vi "NI 5772 (AC) Digitizer(FPGA).vi"() -> ()   [LabVIEW 2020]
doc: "Example Description:\nThis example demonstrates how to enable Time Interleaved Sampling with the NI 5772 adapter module to achieve a sampling rate of 1.6GS/s. This example continuously acquires records of analog input data from the NI 5772 adapter module. It allows you to select an AI channel, trigger type, and record size. This VI must be compiled before it is run. \n\nRunning the VI:\nThis VI must be run from the NI 5772 - Getting Started (Host).vi. Refer to the host VI documentation for steps regarding running and configuring the FPGA VI. \n\nExecution Steps:\nRefer to the Block Diagram of this VI for execution comments."
uses:
  Controls/AI Trigger Type.ctl
  Controls/Aquire State.ctl
  <vilib>/Platform/TimedLoop/XDataNode/timing_clust.ctl
  <vilib>/Platform/TimedLoop/XDataNode/nitl_modes.ctl
  <vilib>/Platform/TimedLoop/XDataNode/wakeup.ctl
  Controls/DigitizerState.ctl
  <instrlib>/_niInstr/Data Trigger/v1/Shared/Public/Edge Configuration Bool.ctl
  <instrlib>/_niInstr/Data Trigger/v1/Shared/Public/Edge Configuration Trigger Slope.ctl
  <vilib>/rvi/Emulation/niFpgaGetClockAttributes.vi
  <vilib>/rvi/Emulation/niFpgaSctlEmulationGetInTimedLoop.vi
  <vilib>/rvi/Emulation/niFpgaEmulationReportErrorSimple.vi
  <vilib>/rvi/eio/common/nirviEmuTemplateMethod_errors.vi
  <vilib>/rvi/Emulation/niFpgaCriticalErrorInLSC.vi
  <instrlib>/_niInstr/Data Trigger/v1/FPGA/Private/Trigger/Edge Boolx1spc.vi
  <vilib>/rvi/Emulation/niFpgaEmulationIsFPGAContextNoSignature.vi
  <vilib>/rvi/errors/niFpgaSetErrorForExecOnDevCompSimple.vi
  <vilib>/rvi/eio/common/nirviEmuReportErrorAndStop.vi
  <vilib>/rvi/DataTransferAndStorage/Container/Common/niFpgaContainerGetUniqueNameForEmu.vi
  <vilib>/rvi/FIFO/Fifo_Resource/nirvififoEmulationSetSize.vi
  <vilib>/rvi/FIFO/Fifo_Resource/nirviFifoEmulationQueueMgr.vi
  <instcachedir>/0/nirviFifoEmulationQueueMgr_E5CAEC123FF24DC58D834DCA3CDAA9B5.lvgen/nirviFifoEmulationQueueMgr_E5CAEC123FF24DC58D834DCA3CDAA9B5_000.vi
  <vilib>/rvi/FIFO/Fifo_Resource/nirvififoEmulationDetermineInputValidOut.vi
  <vilib>/rvi/FIFO/Fifo_Resource/nirvififoEmulationCreateLock.vi
  <vilib>/rvi/Emulation/niFpgaProcessEmulError.vi
  <vilib>/rvi/FIFO/Fifo_Resource/nirvififoEmulationObtainLock.vi
  <vilib>/rvi/FIFO/Fifo_Resource/nirvififoEmulationReleaseLock.vi
  <vilib>/rvi/occurrence/nirviWaitOnOccurrenceBase.vi
  <vilib>/rvi/errors/nirviReportUnexpectedCaseInternalError.vi
  <vilib>/rvi/errors/nirviReportUnexpectedCaseInternalError (U32).vi
  <vilib>/Utility/error.llb/Clear Errors.vi
  <instcachedir>/0/nirviFifoEmulationQueueMgr_E5CAEC123FF24DC58D834DCA3CDAA9B5.lvgen/nirviFifoEmulationQueueMgr_E5CAEC123FF24DC58D834DCA3CDAA9B5_003.vi
  <vilib>/rvi/interface/RandomDataEmulation/niFpgaRandomDataHandleErrors.vi
  <vilib>/eio/EIONode/EIONode.xnode
  <vilib>/Platform/TimedLoop/XDataNode/XDataNode.xnode
  <vilib>/rvi/DataTransferAndStorage/Container/XNode/niFpgaContainer.xnode
  <vilib>/rvi/FIFO/Fifo_Resource/nirvififoEmulationWrite.vi
  <vilib>/rvi/FIFO/Fifo_Resource/nirvififoEmulationRead.vi
  <vilib>/rvi/FIFO/Fifo_Resource/nirvififoEmulationGetNumberOfElementsToRead.vi
  <vilib>/Platform/TimedLoop/XDataNode/XDNodeRunTimeDep.lvlib
  <instrlib>/_niInstr/Data Trigger/v1/FPGA/niInstr Data Trigger v1 FPGA.lvlib
  <instrlib>/_niInstr/Data Trigger/v1/Shared/niInstr Data Trigger v1 Shared.lvlib
  <vilib>/rvi/interface/RandomDataEmulation/nirviRandomDataFpgaReadWriteTemplate.vi
panel:
  out "DMA FIFO Overflow?":bool caption="FIFO Overflow?"
  in  "AvgCount":u16=1
  out "Avg FIFO Overflow?":bool caption="FIFO Overflow?"
  in  "vi/nGenTrig":bool
  in  "TrigIn Simulate":bool
  in  "Delay after Trig [cycles]":u16
  out "TS FIFO In Overflow?":bool caption="FIFO Overflow?"
  in  "Quad Samples Per Trigger":u16=512 caption="Samples Per Trigger" min=1 step=1
  in  "Arm Trigger":bool
  in  "User Command Commit":bool
  in  "User Command":u8
  out "User Command Idle":bool
  out "User Command Status":u8
  in  "User Data 0":u16
  in  "User Data 1":u8
  out "PLL Locked":bool
  out "User Error":bool
  out "Configured?":bool
  in  "Trigger Level":i16
  in  "Trigger Type":T1
  # "Resource Configuration"
  # "Analog Input"
  # "Clock Configuration"
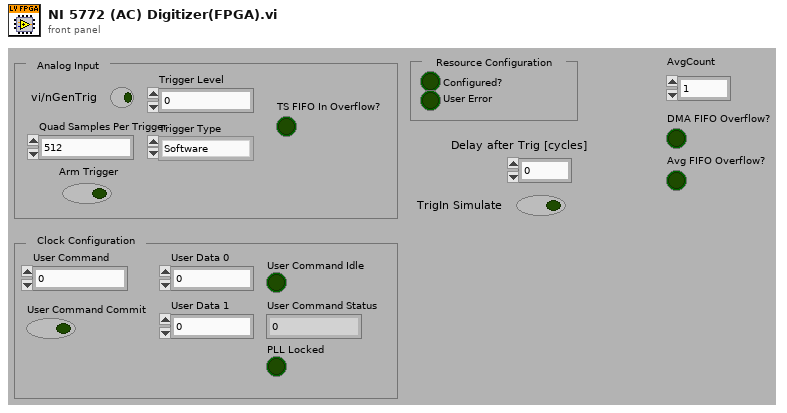
[diagram p1: front panel]
types:
  T1 = typedef "AI Trigger Type.ctl" = enum8{"Software", "Data Edge"}
  T2 = typedef "DigitizerState.ctl" = enum16{"GetData", "Filter", "AverageCountCheck", "SendtoHost", "CompleteScan"}
  T3 = typedef "Aquire State.ctl" = enum8{"Idle", "Wait for Trigger", "Hold Aquire", "Acquire"}
  T4 = typedef "XDNodeRunTimeDep.lvlib/timing_clust.ctl" = cluster{"Expected End [f-1]":u64, "Actual End [f-1]":u64, "Finished Late? [f-1]":bool, "Expected End [i-1]":u64, "Actual End [i-1]":u64, "Finished Late? [i-1]":bool, "Expected Start [i]":u64, "Actual Start [i]":u64, "Expected Start [f]":u64, "Actual Start [f]":u64, "Source Name":string, "Structure Name":string, "Period":i64, "Deadline":i64, "Offset":i64, "Start":i64, "Priority":i32, "Timeout":i32, "Mode":T5, "Wakeup Reason":T6, "Error":errorcluster, "Source Type":string, "Secondary Source Type":string, "Global End Time":u64, "Global Start Time":u64, "Frame Duration":u64, "Iteration Duration":u64, "Assigned CPU":i32, "I/O Scan Engine Mode":u32}
  T5 = typedef "XDNodeRunTimeDep.lvlib/nitl_modes.ctl" = enum32{"No Change", "Process missed periods, maintain original phase", "Discard missed periods, maintain original phase", "Process missed periods, ignore original phase", "Discard missed periods, ignore original phase"}
  T6 = typedef "XDNodeRunTimeDep.lvlib/wakeup.ctl" = enum32{"Normal", "Aborted", "Asynchronous wakeup", "Timing source error", "Timed loop error", "Timeout"}
  T7 = typedef "niInstr Data Trigger v1 Shared.lvlib/Edge Configuration Bool.ctl" = cluster{"trigger slope":T8}
  T8 = typedef "niInstr Data Trigger v1 Shared.lvlib/Edge Configuration Trigger Slope.ctl" = enum8{"Positive", "Negative"}
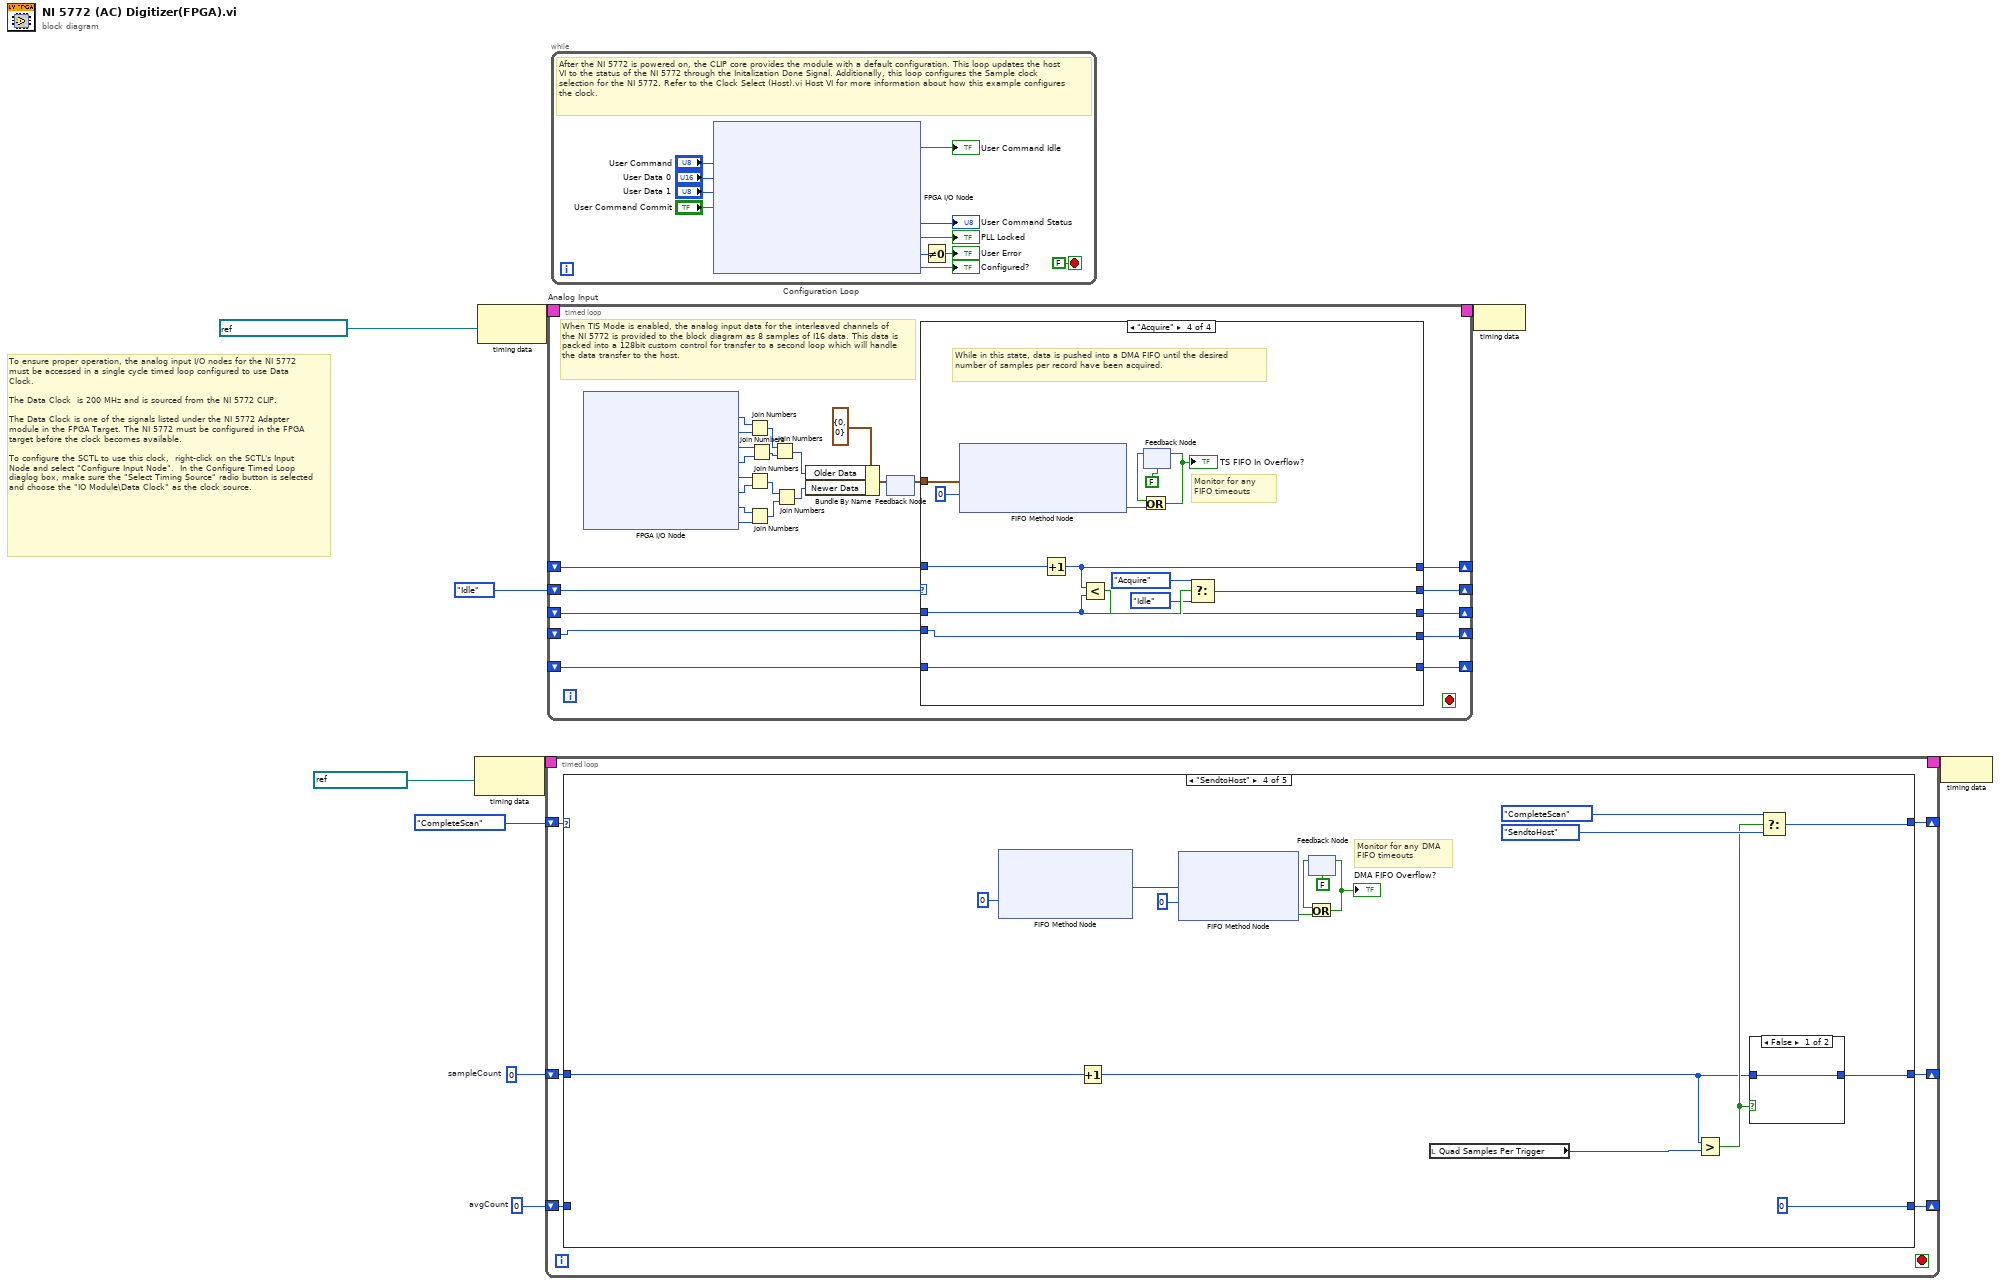
[diagram p0: block diagram]
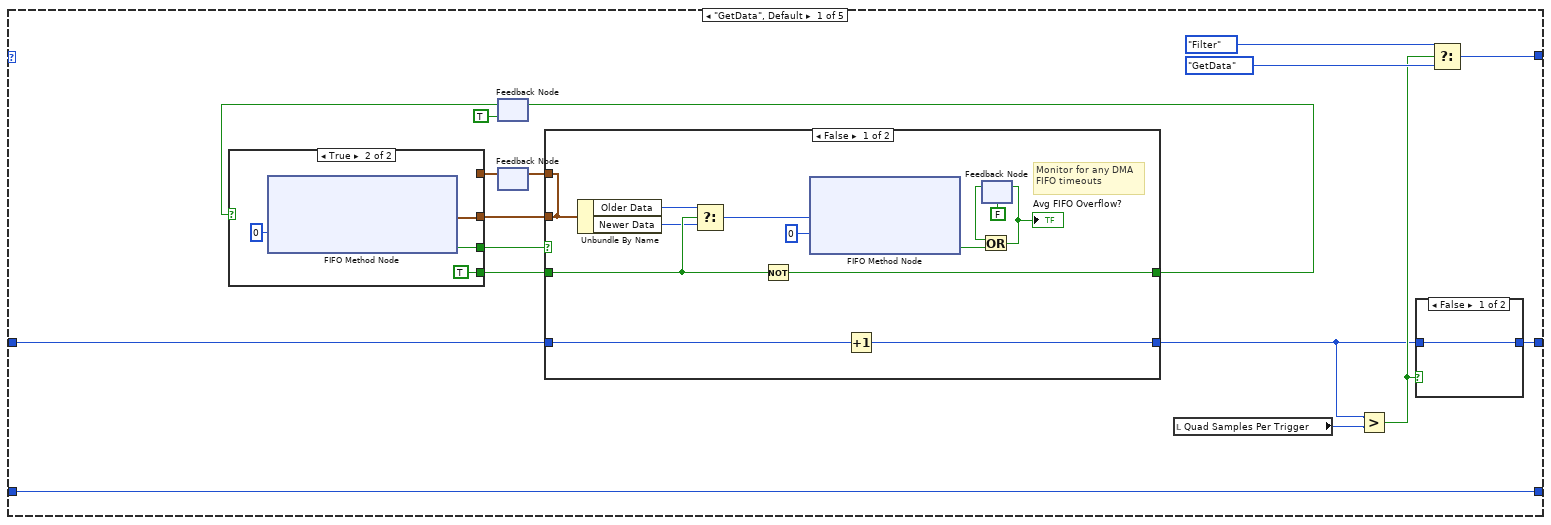
[diagram p2: hidden frame]
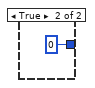
[diagram p3: hidden frame]
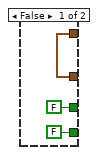
[diagram p4: hidden frame]
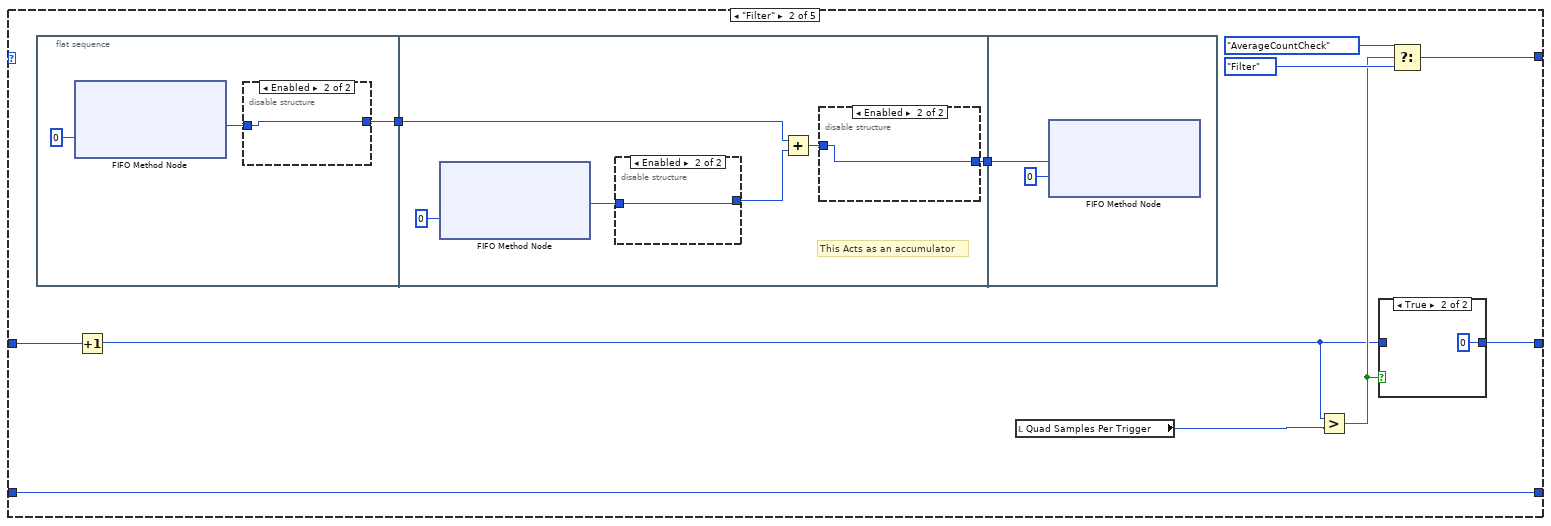
[diagram p6: hidden frame]
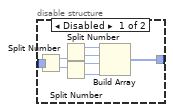
[diagram p7: hidden frame]
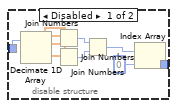
[diagram p8: hidden frame]
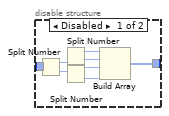
[diagram p9: hidden frame]
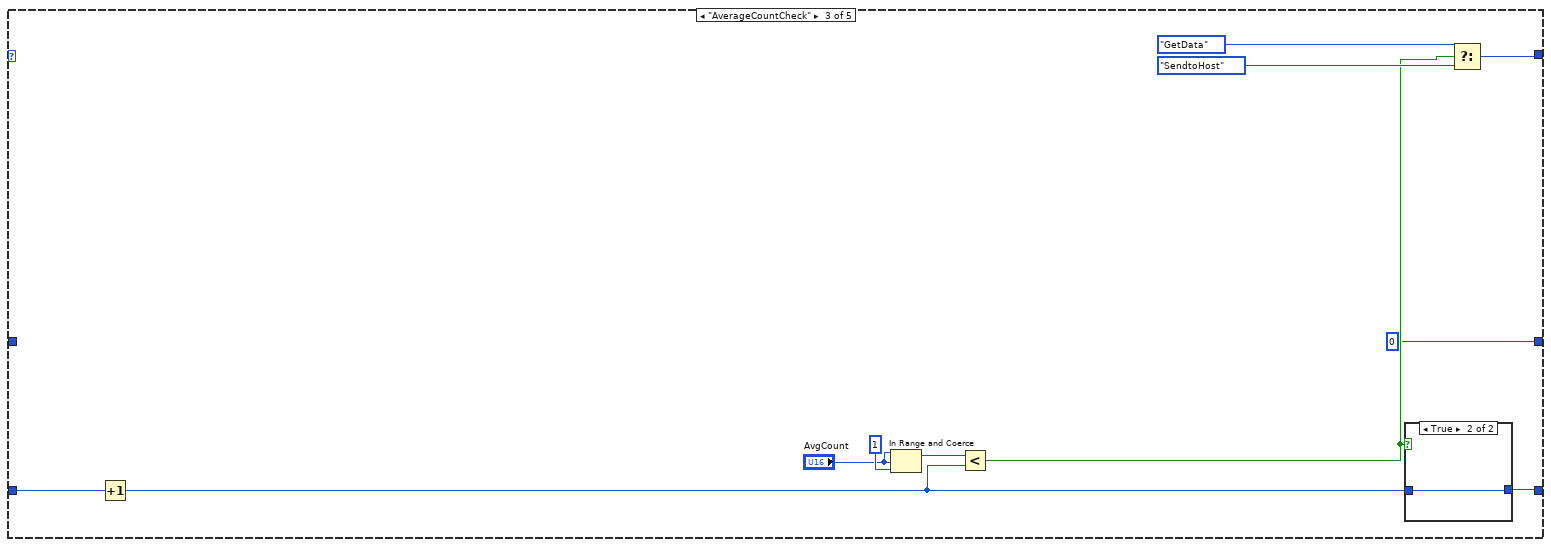
[diagram p11: hidden frame]
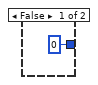
[diagram p12: hidden frame]
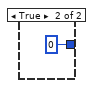
[diagram p13: hidden frame]
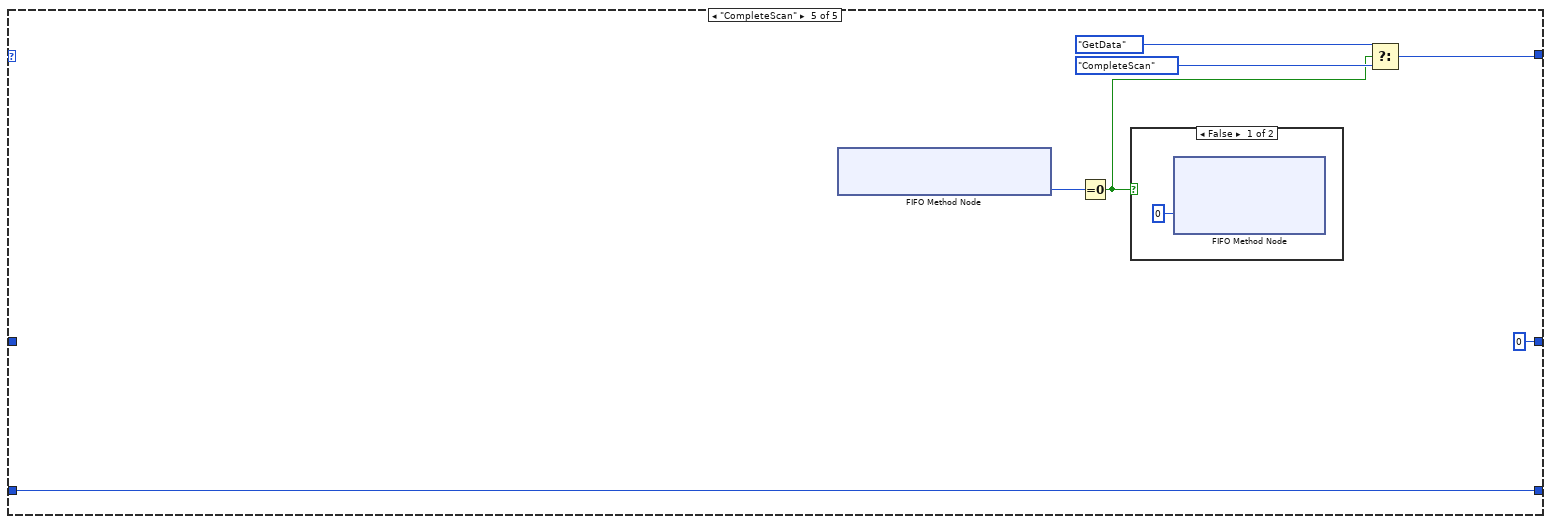
[diagram p14: hidden frame]
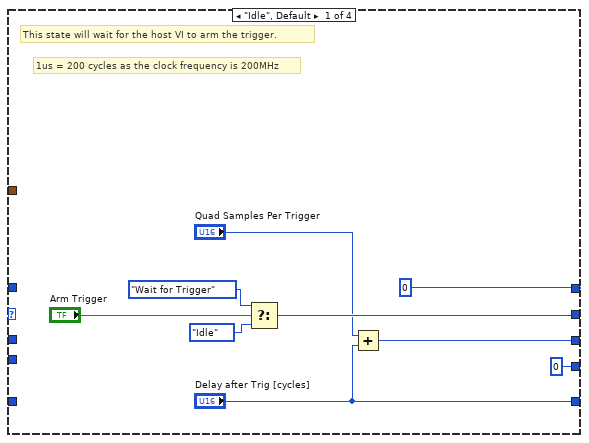
[diagram p16: hidden frame]
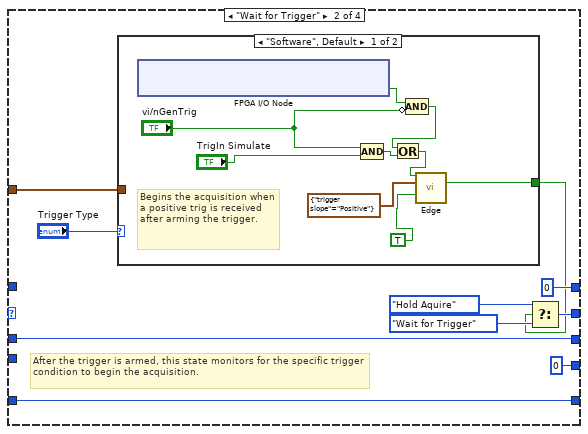
[diagram p17: hidden frame]
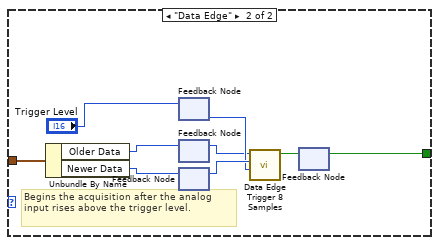
[diagram p18: hidden frame]
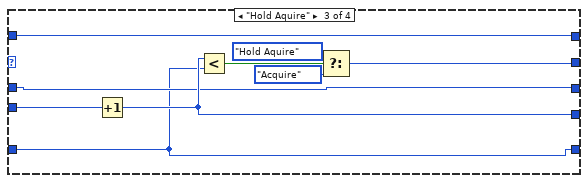
[diagram p19: hidden frame]
diagram:
  w1 = u16 0  # avgCount
  w2 = u32 0  # sampleCount
  # "To ensure proper operation, the analog input I/O nodes for the NI 5772 must be accessed in a single cycle timed loop configured to use Data Clock. \n\nThe Data Clock  is 200 MHz and is sourced from the NI 5772 CLIP.\n\nThe Data Clock is one of the signals listed under the NI 5772 Adapter module in the FPGA Target. The NI 5772 must be configured in the FPGA target before the clock becomes available. \n\nTo configure the SCTL to use this clock,  right-click on the SCTL's Input Node and select \"Configure Input Node\".  In the Configure Timed Loop diaglog box, make sure the \"Select Timing Source\" radio button is selected and choose the \"IO Module\\Data Clock\" as the clock source."
  n1 = node-c288(refnum<k21> "100 MHz Clock" ("Source Name")) -> (w6:T4)
  n2 = node-c288(refnum<k21> "IO Module\\Data Clock" ("Source Name")) -> (w10:T4)
  n3 = timed-loop {
    timing: w6 -> [_]
    timing-out: [_] -> w5
    shift-right: [w14] -> _
    shift-left: w2 -> [w15]
    shift-right: [w13] -> _
    shift-left: DigitizerState."CompleteScan" -> [w16]
    shift-right: [w11] -> _
    shift-left: w1 -> [w12]
    stop <- _ stop-if-true
    n4 = case shown="\"SendtoHost\"" w16 {
      tunnel: w15 -> [w25 w69 _ w127 _]
      tunnel: [w18 w64 u32 0 ("sampleCount") w128 u32 0 ("sampleCount")] -> w14
      tunnel: [w23 w65 w116 w129 w146] -> w13
      tunnel: w12 -> [w17 w61 w122 _ w149]
      tunnel: [w17 w61 w115 u16 0 ("sampleCount") w149] -> w11
      frame "GetData", Default {
        n5 = feedback #1(TRUE ("Timed Out?")) -> (w32:bool)
        n6 = feedback #2() -> (w31:cluster{"Older Data":u64, "Newer Data":u64})  [unwired: 1 in]
        n7 = case shown="True" w32 {
          tunnel: [w36 w39] -> w29
          tunnel: [FALSE ("Timed Out?") w40] -> w28
          tunnel: [FALSE ("Timed Out?") TRUE ("Timed Out?")] -> w27
          tunnel: w31 -> [w36 _]
          frame False {
          }
          frame True {
            n8 = xnode ("FIFO Method Node")("Timeout"=0) -> ("Element"=w39:cluster{"Older Data":u64, "Newer Data":u64}, "Timed Out?"=w40:bool)  [unwired: 1 in, 1 out]
          }
        }
        n9 = case shown="False" w28 {
          tunnel: [w53 w58] -> w26
          tunnel: w27 -> [w54 w58]
          tunnel: w29 -> [w52 w57]
          tunnel: [w52 w57] -> w30
          tunnel: [w43 w56] -> w19
          tunnel: w25 -> [w44 w56]
          frame False {
            # "Monitor for any DMA FIFO timeouts"
            n10 = Unbundle By Name(w52) -> ("Older Data"=w55:u64, "Newer Data"=w51:u64)
            n11 = Select(t=w55, s=w54, f=w51) -> (s? t:f=w45:u64)
            n12 = Not(x=w54) -> (.not. x?=w53:bool)
            n13 = xnode ("FIFO Method Node")("Element"=w45, "Timeout"=0) -> ("Timed Out?"=w49:bool)  [unwired: 1 in, 1 out]
            n14 = Increment(x=w44) -> (x+1=w43:u32)
            n15 = feedback #3(FALSE) -> (w46:bool)
            n16 = Or(x=w46, y=w49) -> (x .or. y?=w48:bool)
            "Avg FIFO Overflow?" <- w48
            n17 = feedback-in #3(w48) -> ()
          }
          frame True {
          }
        }
        n18 = feedback-in #1(w26) -> ()
        n19 = feedback-in #2(w30) -> ()
        n20 = local read "Quad Samples Per Trigger"() -> (w21:u16)
        n21 = Greater?(x=w19, y=w21) -> (0:w20:bool)
        n22 = case shown="False" w20 {
          tunnel: w19 -> [w34 _]
          tunnel: [w34 u32 0 ("sampleCount")] -> w18
          frame False {
          }
          frame True {
          }
        }
        n23 = Select(t=DigitizerState."Filter", s=w20, f=DigitizerState."GetData") -> (s? t:f=w23:T2)
      }
      frame "Filter" {
        n24 = flat-sequence {
          tunnel: [w70] -> w59
          tunnel: [w85] -> w60
          tunnel: w59 -> [w84]
          tunnel: w60 -> [w108]
          frame #0 {
            n25 = xnode ("FIFO Method Node")("Timeout"=0) -> ("Element"=w72:u64)  [unwired: 1 in, 2 out]
            n26 = disable-structure shown="Enabled" {
              disable-tunnel: w72 -> [w80 w81]
              disable-tunnel: [w76 w81] -> w70
              frame Disabled {
                n27 = Split Number(x=w80) -> (hi(x)=w78:u32, lo(x)=w77:u32)
                n28 = Split Number(x=w78) -> (hi(x)=w79:u16, lo(x)=w75:u16)
                n29 = Split Number(x=w77) -> (hi(x)=w74:u16, lo(x)=w73:u16)
                n30 = Build Array(w79, w75, w74, w73) -> (w76:u16[])
              }
              frame Enabled {
              }
            }
          }
          frame #1 {
            # "This Acts as an accumulator"
            n31 = xnode ("FIFO Method Node")("Timeout"=0) -> ("Element"=w83:u64)  [unwired: 1 in, 2 out]
            n32 = disable-structure shown="Enabled" {
              disable-tunnel: w83 -> [w100 w107]
              disable-tunnel: [w99 w107] -> w82
              frame Disabled {
                n33 = Split Number(x=w100) -> (hi(x)=w105:u32, lo(x)=w104:u32)
                n34 = Split Number(x=w105) -> (hi(x)=w106:u16, lo(x)=w103:u16)
                n35 = Split Number(x=w104) -> (hi(x)=w102:u16, lo(x)=w101:u16)
                n36 = Build Array(w106, w103, w102, w101) -> (w99:u16[])
              }
              frame Enabled {
              }
            }
            n37 = Add(x=w84, y=w82) -> (x+y=w86:u64)
            n38 = disable-structure shown="Enabled" {
              disable-tunnel: w86 -> [w91 w98]
              disable-tunnel: [w88 w98] -> w85
              frame Disabled {
                n39 = Decimate 1D Array(w91) -> (w97:dbl[], w96:dbl[], w95:dbl[], w92:dbl[])
                n40 = Join Numbers(hi=w97, lo=w96) -> ((hi.lo)=w94:u32)
                n41 = Join Numbers(hi=w95, lo=w92) -> ((hi.lo)=w93:u32)
                n42 = Join Numbers(hi=w94, lo=w93) -> ((hi.lo)=w89:u64)
                n43 = Index Array(array=w89, index=0) -> (element=w88)
              }
              frame Enabled {
              }
            }
          }
          frame #2 {
            n44 = xnode ("FIFO Method Node")("Element"=w108, "Timeout"=0) -> ()  [unwired: 1 in, 2 out]
          }
        }
        n45 = Increment(x=w69) -> (x+1=w63:u32)
        n46 = local read "Quad Samples Per Trigger"() -> (w62:u16)
        n47 = Greater?(x=w63, y=w62) -> (0:w66:bool)
        n48 = case shown="True" w66 {
          tunnel: w63 -> [w110 _]
          tunnel: [w110 u32 0 ("sampleCount")] -> w64
          frame False {
          }
          frame True {
          }
        }
        n49 = Select(t=DigitizerState."AverageCountCheck", s=w66, f=DigitizerState."Filter") -> (s? t:f=w65:T2)
      }
      frame "AverageCountCheck" {
        n50 = Increment(x=w122) -> (x+1=w114:u16)
        n51 = In Range and Coerce(upper limit="AvgCount", x="AvgCount", lower limit=u16 1) -> (coerced(x)=w119:u16)  [unwired: 1 out]
        n52 = Less?(x=w119, y=w114) -> (x < y?=w113:bool)
        n53 = case shown="True" w113 {
          tunnel: [u16 0 ("sampleCount") w124] -> w115
          tunnel: w114 -> [_ w124]
          frame False {
          }
          frame True {
          }
        }
        n54 = Select(t=DigitizerState."GetData", s=w113, f=DigitizerState."SendtoHost") -> (s? t:f=w116:T2)
      }
      frame "SendtoHost" {
        # "Monitor for any DMA FIFO timeouts"
        n55 = xnode ("FIFO Method Node")("Timeout"=0) -> ("Element"=w134:u64)  [unwired: 1 in, 2 out]
        n56 = Increment(x=w127) -> (x+1=w126:u32)
        n57 = xnode ("FIFO Method Node")("Element"=w134, "Timeout"=0) -> ("Timed Out?"=w138:bool)  [unwired: 1 in, 1 out]
        n58 = feedback #4(FALSE) -> (w135:bool)
        n59 = Or(x=w135, y=w138) -> (x .or. y?=w137:bool)
        "DMA FIFO Overflow?" <- w137
        n60 = feedback-in #4(w137) -> ()
        n61 = local read "Quad Samples Per Trigger"() -> (w130:u16)
        n62 = Greater?(x=w126, y=w130) -> (0:w131:bool)
        n63 = case shown="False" w131 {
          tunnel: w126 -> [w141 _]
          tunnel: [w141 u32 0 ("sampleCount")] -> w128
          frame False {
          }
          frame True {
          }
        }
        n64 = Select(t=DigitizerState."CompleteScan", s=w131, f=DigitizerState."SendtoHost") -> (s? t:f=w129:T2)
      }
      frame "CompleteScan" {
        n65 = xnode ("FIFO Method Node")() -> ("Number of Elements to Read"=w145:u32)  [unwired: 1 in, 1 out]
        n66 = Equal To 0?(x=w145) -> (x = 0?=w144:bool)
        n67 = case shown="False" w144 {
          frame False {
            n68 = xnode ("FIFO Method Node")("Timeout"=0) -> ()  [unwired: 1 in, 3 out]
          }
          frame True {
          }
        }
        n69 = Select(t=DigitizerState."GetData", s=w144, f=DigitizerState."CompleteScan") -> (s? t:f=w146:T2)
      }
    }
  }
  n70 = timed-loop "Analog Input" {
    timing: w10 -> [_]
    timing-out: [_] -> w9
    shift-right: [w178] -> _
    shift-left: Aquire_State."Idle" ("Acquire State") -> [w168]
    shift-right: [w179] -> _
    shift-left: _ -> [w169]
    shift-right: [w177] -> _
    shift-left: _ -> [w167]
    shift-right: [w156] -> _
    shift-left: _ -> [w155]
    shift-right: [w153] -> _
    shift-left: _ -> [w154]
    stop <- _ stop-if-true
    # "When TIS Mode is enabled, the analog input data for the interleaved channels of the NI 5772 is provided to the block diagram as 8 samples of I16 data. This data is packed into a 128bit custom control for transfer to a second loop which will handle the data transfer to the host."
    n71 = xnode "FPGA I/O Node"() -> ("IO Module\\AI 1 Data N-3"=w160:i16, "IO Module\\AI 0 Data N-3"=w159:i16, "IO Module\\AI 1 Data N-2"=w158:i16, "IO Module\\AI 0 Data N-2"=w157:i16, "IO Module\\AI 1 Data N-1"=w161:i16, "IO Module\\AI 0 Data N-1"=w162:i16, "IO Module\\AI 1 Data N"=w163:i16, "IO Module\\AI 0 Data N"=w164:i16)  [unwired: 8 in, 8 out]
    n72 = Join Numbers(hi=w160, lo=w159) -> ((hi.lo)=w172:u32)
    n73 = Join Numbers(hi=w161, lo=w162) -> ((hi.lo)=w173:u32)
    n74 = Join Numbers(hi=w163, lo=w164) -> ((hi.lo)=w175:u32)
    n75 = Join Numbers(hi=w158, lo=w157) -> ((hi.lo)=w174:u32)
    n76 = Join Numbers(hi=w172, lo=w174) -> ((hi.lo)=w166:u64)
    n77 = Join Numbers(hi=w173, lo=w175) -> ((hi.lo)=w165:u64)
    n78 = Bundle By Name(cluster=cluster{"Older Data":u64, "Newer Data":u64} {"Older Data"=0, "Newer Data"=0} ("Element"), "Older Data"=w166, "Newer Data"=w165) -> (w170:cluster{"Older Data":u64, "Newer Data":u64})
    n79 = feedback #5() -> (w176:cluster{"Older Data":u64, "Newer Data":u64})  [unwired: 1 in]
    n80 = feedback-in #5(w170) -> ()
    n81 = case shown="\"Acquire\"" w168 {
      tunnel: [u16 0 u16 0 w219 w240] -> w179
      tunnel: w169 -> [_ _ w219 w239]
      tunnel: [w185 w193 w222 w237] -> w178
      tunnel: [w182 w197 w218 w234] -> w177
      tunnel: w167 -> [_ w197 w218 w234]
      tunnel: w176 -> [_ w196 _ w233]
      tunnel: [u16 0 ("Delay after Trig [cycles]") u16 0 ("Delay after Trig [cycles]") w220 w227] -> w156
      tunnel: w155 -> [_ _ w221 w227]
      tunnel: w154 -> [_ w189 w217 w226]
      tunnel: ["Delay after Trig [cycles]" w189 w217 w226] -> w153
      frame "Idle", Default {
        # "1us = 200 cycles as the clock frequency is 200MHz"
        # "This state will wait for the host VI to arm the trigger."
        n82 = Select(t=Aquire_State."Wait for Trigger" ("Acquire State"), s="Arm Trigger", f=Aquire_State."Idle" ("Acquire State")) -> (s? t:f=w185:T3)
        n83 = Add(x="Quad Samples Per Trigger", y="Delay after Trig [cycles]") -> (x+y=w182:u16)
      }
      frame "Wait for Trigger" {
        # "After the trigger is armed, this state monitors for the specific trigger condition to begin the acquisition."
        n84 = case shown="\"Software\", Default" "Trigger Type" {
          tunnel: w196 -> [_ w216]
          tunnel: [w207 w208] -> w191
          frame "Software", Default {
            # "Begins the acquisition when a positive trig is received after arming the trigger."
            n85 = xnode "FPGA I/O Node"() -> ("IO Module\\Asynchronous Trigger Input"=w203:bool)  [unwired: 1 in, 1 out]
            n86 = Compound Arithmetic op=AND("vi/nGenTrig", "TrigIn Simulate") -> (w199:bool)
            n87 = Compound Arithmetic op=AND(w203, invert "vi/nGenTrig") -> (w202:bool)
            n88 = Or(x=w202, y=w199) -> (x .or. y?=w204:bool)
            n89 = call-poly <instrlib>:"Edge.vi"("data in"=w204, "configuration"=T7 {"trigger slope"=enum."Positive"}, "input valid"=TRUE) -> ("trigger"=w207:bool)  [unwired: 7 in, 5 out]
          }
          frame "Data Edge" {
            # "Begins the acquisition after the analog input rises above the trigger level."
            n90 = Unbundle By Name(w216) -> ("Older Data"=w214:u64, "Newer Data"=w212:u64)
            n91 = feedback-in #6("Trigger Level") -> ()
            n92 = feedback #6() -> (w210:i16)  [unwired: 1 in]
            n93 = feedback-in #7(w214) -> ()
            n94 = feedback #7() -> (w209:u64)  [unwired: 1 in]
            n95 = feedback-in #8(w212) -> ()
            n96 = feedback #8() -> (w211:u64)  [unwired: 1 in]
            n97 = call "Data Edge Trigger 8 Samples.vi"("Trigger Level"=w210, "Newer Data In"=w211, "Older Data In"=w209) -> ("Trigger"=w215:bool)  [unwired: 8 in]
            n98 = feedback-in #9(w215) -> ()
            n99 = feedback #9() -> (w208:bool)  [unwired: 1 in]
          }
        }
        n100 = Select(t=Aquire_State."Hold Aquire" ("Acquire State"), s=w191, f=Aquire_State."Wait for Trigger") -> (s? t:f=w193:T3)
      }
      frame "Hold Aquire" {
        n101 = Increment(x=w221) -> (x+1=w220:u16)
        n102 = Less?(x=w220, y=w217) -> (x < y?=w225:bool)
        n103 = Select(t=Aquire_State."Hold Aquire" ("Acquire State"), s=w225, f=Aquire_State."Acquire" ("Acquire State")) -> (s? t:f=w222:T3)
      }
      frame "Acquire" {
        # "Monitor for any  FIFO timeouts"
        # "While in this state, data is pushed into a DMA FIFO until the desired number of samples per record have been acquired."
        n104 = xnode ("FIFO Method Node")("Element"=w233, "Timeout"=0) -> ("Timed Out?"=w228:bool)  [unwired: 1 in, 1 out]
        n105 = Increment(x=w239) -> (x+1=w240:u16)
        n106 = Less?(x=w240, y=w234) -> (x < y?=w238:bool)
        n107 = feedback #10(FALSE) -> (w229:bool)
        n108 = Or(x=w229, y=w228) -> (x .or. y?=w230:bool)
        "TS FIFO In Overflow?" <- w230
        n109 = feedback-in #10(w230) -> ()
        n110 = Select(t=Aquire_State."Acquire" ("Acquire State"), s=w238, f=Aquire_State."Idle" ("Acquire State")) -> (s? t:f=w237:T3)
      }
    }
  }
  n111 = while "Configuration Loop" {
    stop <- FALSE stop-if-true
    # "After the NI 5772 is powered on, the CLIP core provides the module with a default configuration. This loop updates the host VI to the status of the NI 5772 through the Initalization Done Signal. Additionally, this loop configures the Sample clock selection for the NI 5772. Refer to the Clock Select (Host).vi Host VI for more information about how this example configures the clock."
    n112 = xnode "FPGA I/O Node"("IO Module\\User Command"="User Command", "IO Module\\User Data 0"="User Data 0", "IO Module\\User Data 1"="User Data 1", "IO Module\\User Command Commit"="User Command Commit") -> ("IO Module\\User Command Idle"=→"User Command Idle":bool, "IO Module\\User Command Status"=→"User Command Status":u8, "IO Module\\PLL Locked"=→"PLL Locked":bool, "IO Module\\User Error"=w248:u8, "IO Module\\Initialization Done"=→"Configured?":bool)  [unwired: 9 in, 9 out]
    n113 = Not Equal To 0?(x=w248) -> (x != 0?=→"User Error":bool)
  }
  n114 = node-c288(w9) -> ()
  n115 = node-c288(w5) -> ()
